vi "Detector Update FITS Header.vi"(8 "error in (no error)":errorcluster, 9 "Offsets":u16[](array[numeric]) format="%.0x", 10 "FITS Detector Settings":T1, 11 "FITS File":path) -> (0 "error out":errorcluster)   [LabVIEW 2020]
uses:
  RIMAS Observation Config.ctl
panel:
  out "text":string[](array[string])
  # "sec"
  # "sec"
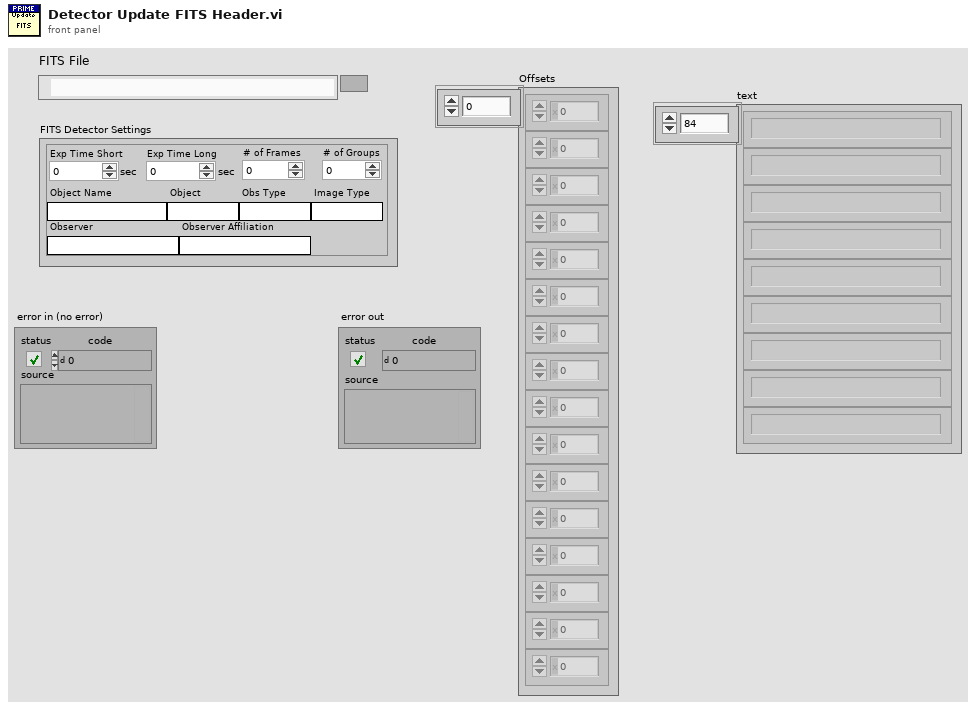
[diagram p1: front panel]
types:
  T1 = typedef "RIMAS Observation Config.ctl" = cluster{"Exp Time Short":dbl, "# of Frames":dbl, "Exp Time Long":dbl, "# of Groups":dbl, "Object Name":string, "Object":string, "Obs Type":string, "Image Type":string, "Observer":string, "Observer Affiliation":string}
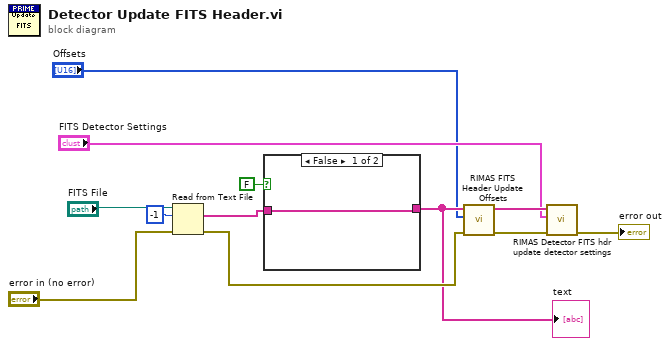
[diagram p0: block diagram]
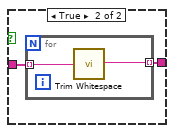
[diagram p2: hidden frame]
diagram:
  n1 = Read from Text File(file (use dialog)="FITS File", count=-1, error in="error in (no error)") -> (text=w8:string[], error out=w11:errorcluster)  [unwired: 1 in, 2 out]
  n2 = case shown="False" FALSE {
    tunnel: w8 -> [w13 w15]
    tunnel: [w13 w14] -> w7
    frame False {
    }
    frame True {
      n3 = for {
        tunnel: w15 -> [w16] mode=indexing
        tunnel: [w17] -> w14 mode=indexing
        n4 = call <vilib>:"Trim Whitespace.vi"("string"=w16) -> ("trimmed string"=w17:string)  [unwired: 1 in]
      }
    }
  }
  "text" <- w7
  n5 = call "RIMAS FITS Header Update Offsets.vi"("Error In"=w11, "Offsets"="Offsets", "header file"=w7) -> ("Error Out"=w10:errorcluster, "updated hdr file"=w9:string[])  [unwired: 7 in]
  n6 = call "RIMAS Detector FITS hdr update detector settings.vi"("Error In"=w10, "FITS Detector Settings"="FITS Detector Settings", "fits hdr"=w9) -> ("Error Out"=→"error out":errorcluster)  [unwired: 7 in, 1 out]
